vi "MotorTest.vi"() -> ()   [LabVIEW 2016]
panel:
  in  "State":dbl
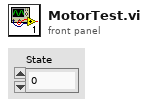
[diagram p1: front panel]
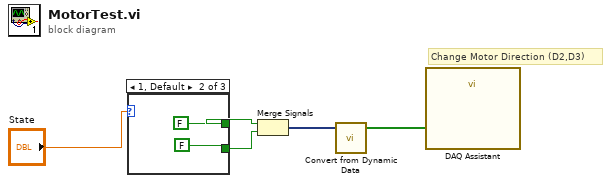
[diagram p0: block diagram]
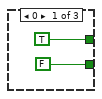
[diagram p2: hidden frame]
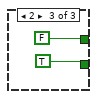
[diagram p3: hidden frame]
diagram:
  # "Change Motor Direction (D2,D3)"
  n1 = case shown="1, Default" "State" {
    tunnel: [TRUE FALSE FALSE] -> w3
    tunnel: [FALSE FALSE TRUE] -> w2
    frame 0 {
    }
    frame 1, Default {
    }
    frame 2 {
    }
  }
  n2 = Merge Signals(w3, w2) -> (w5:dynamicdata)
  n3 = call "Convert from Dynamic Data"("Dynamic Data Type"=w5) -> ("Array"=w4:bool[])  [unwired: 3 in]
  n4 = call "DAQ Assistant"("data"=w4) -> ()  [unwired: 17 in, 2 out]
